vi "ex2.vi"() -> ()   [LabVIEW 2022 SP3]
uses:
  <vilib>/numeric/Random Number (Range) DBL.vi
panel:
  in  "Noises Amplitude":dbl
  out "Waveform Chart":cluster{dbl, "Discrimination level":dbl}(graph)
  in  "Discrimination level":dbl
  out "LED":bool
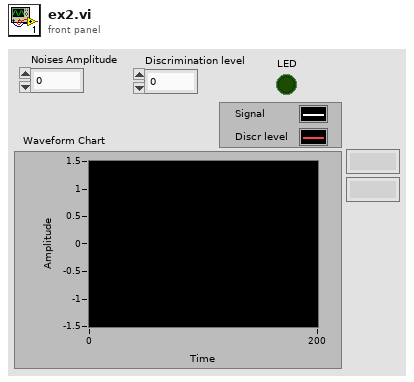
[diagram p1: front panel]
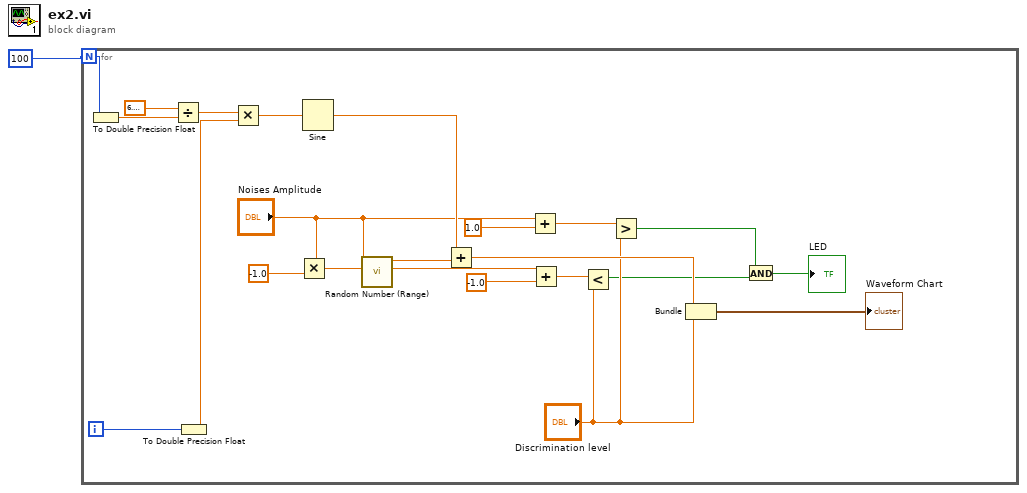
[diagram p0: block diagram]
diagram:
  n1 = for {
    N: 100 -> [w2]
    i -> [w21]
    n2 = To Double Precision Float(number=w2) -> (double precision float=w19:dbl)
    n3 = Divide(x=6.283185307179586, y=w19) -> (x/y=w22:dbl)
    n4 = To Double Precision Float(number=w21) -> (double precision float=w20:dbl)
    n5 = Multiply(x=w22, y=w20) -> (x*y=w16:dbl)
    n6 = Multiply(x="Noises Amplitude", y=-1.0) -> (x*y=w10:dbl)
    n7 = Sine(x=w16) -> (sin(x)=w13:dbl)
    n8 = call-poly <vilib>:"Random Number (Range).vi"("lower bound (0)"=w10, "upper bound (100)"="Noises Amplitude") -> ("number"=w15:dbl)  [unwired: 9 in]
    n9 = Add(x=w13, y=w15) -> (x+y=w14:dbl)
    n10 = Add(x="Noises Amplitude", y=1.0) -> (x+y=w8:dbl)
    n11 = Add(x=w10, y=-1.0) -> (x+y=w7:dbl)
    n12 = Less?(x=w7, y="Discrimination level") -> (x < y?=w4:bool)
    n13 = Greater?(x=w8, y="Discrimination level") -> (0:w5:bool)
    n14 = Bundle(w14, "Discrimination level"="Discrimination level") -> (→"Waveform Chart":cluster{dbl, "Discrimination level":dbl})  [unwired: 1 in]
    n15 = And(x=w5, y=w4) -> (x .and. y?=→"LED":bool)
  }
